vi "Ctor.vi"(8 "error in (no error)":errorcluster) -> (0 "error out":errorcluster, 3 "LabBOT out":refnum<class "LabBOT.lvclass">)   [LabVIEW 2020, in "Rover.lvlib" / "LabBOT.lvclass"]
uses:
  LabBOT.lvclass
  <vilib>/Instr/_visa.llb/VISA Find Search Mode.ctl
  bno055/BNO055/BNO055/Operating Mode.ctl
  LabBOT.lvclass/LabBOT.ctl
  <vilib>/MakerHub/LINX/Public/Utilities/Open Local.vi
  <vilib>/MakerHub/LINX/LMH-LINX.lvlib
  Rover/Rover.lvclass
  bno055/BNO055/BNO055/BNO055.lvclass
  nmea/nmea/VISA GPS/VISA GPS.lvclass
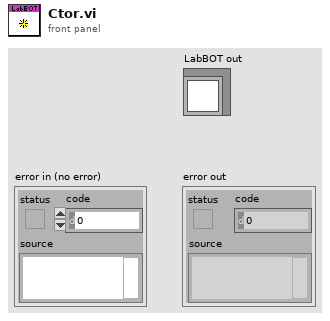
[diagram p1: front panel]
types:
  T1 = typedef "VISA Find Search Mode.ctl" = u32
  T2 = typedef "LMH-LINX.lvlib/LINX Ref.ctl" = cluster{"IO":T3, "Interface":T4, "LINX Device Config":T5}
  T3 = typedef "LMH-LINX.lvlib/Platform.ctl" = enum16{"Remote", "Local"}
  T4 = typedef "LMH-LINX.lvlib/Interface.ctl" = enum16{"Serial", "TCP"}
  T5 = typedef "LMH-LINX.lvlib/Device.lvlib/LINX Device Config.ctl" = cluster{"Interface":T4, "COM Port":refnum<visa-resource-name>, "TCP Configuration":T6, "Device Family":u8, "Device ID":u8, "Device Name":string, "TCP Ref":refnum<k5>, "Channels":T7}
  T6 = typedef "LMH-LINX.lvlib/Device.lvlib/TCP Config.ctl" = cluster{"IP Address":string, "Port":u16}
  T7 = typedef "LMH-LINX.lvlib/Channels.ctl" = cluster{"DI":u8[], "DO":u8[], "AI":u8[], "AO":u8[], "PWM":u8[], "QE":u8[], "UART":u8[], "I2C 2":u8[], "SPI":u8[], "CAN":u8[], "Servo":u8[], "AI Ref (V)":dbl, "AI Resolution (Bits)":u8, "AO Ref (V)":dbl, "AO Resolution (Bits)":u8}
  T8 = typedef "BNO055.lvlib/BNO055.lvclass/Operating Mode.ctl" = enum8{"Config", "Acc Only", "Mag Only", "Gyr Only", "Acc Mag", "Acc Gyr", "Mag Gyr", "AccMagGyr", "IMU", "Compass", "Mag4Gyr", "NDOF FMC Off", "NDOF"}
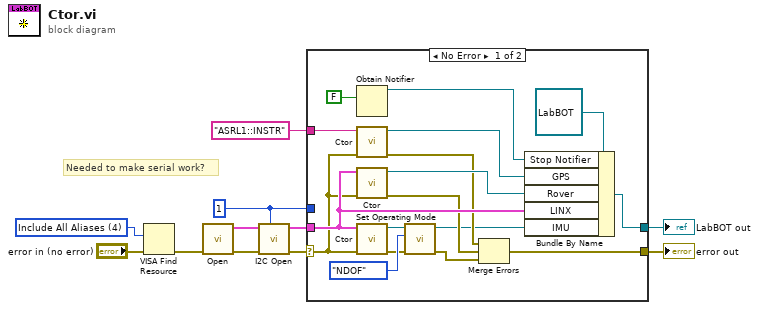
[diagram p0: block diagram]
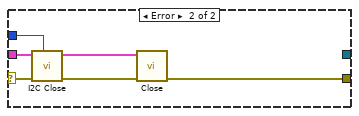
[diagram p2: hidden frame]
diagram:
  w4 = T1 4 items=["Canonical Names Only"=0, "Aliases Only"=2, "Include Matching Aliases"=3, "Include All Aliases"=4] ("Search Mode")
  w5 = u8 1 ("I2C Channel (0)")
  # "Needed to make serial work?"
  n1 = VISA Find Resource(8:"error in (no error)", 10:w4) -> (0:w2:errorcluster)  [unwired: 1 in, 2 out]
  n2 = call-poly <vilib>:"Open.vi"("Error In"=w2) -> ("Error Out"=w9:errorcluster, "LINX Resource"=w8:T2)  [unwired: 8 in, 1 out]
  n3 = call <vilib>:"I2C Open.vi"("I2C Channel (0)"=w5, "Error In"=w9, "LINX Resource"=w8) -> ("Error Out"=w11:errorcluster, "LINX Resource"=w7:T2)  [unwired: 7 in]
  n4 = case shown="No Error" w11 {
    selector: w11 -> [w22 w33]
    tunnel: [w27 _] -> w10
    tunnel: w7 -> [w25 w34]
    tunnel: [w19 w29] -> w6
    tunnel: w5 -> [_ w32]
    tunnel: "ASRL1::INSTR" -> [w24 _]
    frame No Error {
      n5 = Obtain Notifier(notification data type=FALSE) -> (notifier out=w12:refnum<notifier>)  [unwired: 3 in, 2 out]
      n6 = call "Ctor.vi"("error in (no error)"=w22, "VISA Port"=w24) -> ("error out"=w20:errorcluster, "VISA GPS out"=w23:refnum<class "VISA GPS.lvclass">)  [unwired: 8 in]
      n7 = call "Ctor.vi"("error in (no error)"=w22, "LINX Resource"=w25) -> ("error out"=w21:errorcluster, "Rover out"=w26:refnum<class "Rover.lvclass">)  [unwired: 8 in]
      n8 = call "Ctor.vi"("error in (no error)"=w22, "LINX Resource"=w25) -> ("error out"=w16:errorcluster, "BNO055 out"=w17:refnum<class "BNO055.lvclass">)  [unwired: 7 in, 1 out]
      n9 = call "Set Operating Mode.vi"("error in (no error)"=w16, "Operating Mode"=Operating_Mode."NDOF", "BNO055 in"=w17) -> ("error out"=w15:errorcluster, "BNO055 out"=w14:refnum<class "BNO055.lvclass">)  [unwired: 7 in]
      n10 = Merge Errors(w20, w21, w15) -> (w19:errorcluster)
      n11 = Bundle By Name(cluster=refnum<class "LabBOT.lvclass"> refnum ("LabBOT in"), "Stop Notifier"=w12, "GPS"=w23, "Rover"=w26, "LINX"=w25, "IMU"=w14) -> (w27:refnum<class "LabBOT.lvclass">)
    }
    frame Error {
      n12 = call <vilib>:"I2C Close.vi"("I2C Channel (0)"=w32, "Error In"=w33, "LINX Resource"=w34) -> ("Error Out"=w30:errorcluster, "LINX Resource"=w31:T2)  [unwired: 7 in]
      n13 = call <vilib>:"Close.vi"("Error In"=w30, "LINX Resource"=w31) -> ("Error Out"=w29:errorcluster)  [unwired: 9 in]
    }
  }
  "error out" <- w6
  "LabBOT out" <- w10
